vi "CH0_write_byte_data_into_mem.vi"(0 "MB data":u8, 1 "UB data":u8, 3 "USB Interface Name":refnum<visa-resource-name>="COM3", 4 "HB data":u8, 5 "LB data":u8, 6 "MB address":string, 7 "HB address":string, 9 "WRITE DATA":bool, 10 "Input buffer size":u32=16384, 11 "LB address":string, 12 "UB address":string, 13 "error in (no error)":errorcluster) -> (14 "MB data string":string, 15 "UB data string":string, 17 "error out":errorcluster, 18 "HB data string":string, 19 "LB data string":string)   [LabVIEW 2012]
panel:
  out "T command Bytes sent 4":dbl
  out "T command Bytes sent 3":dbl
  out "T command Bytes sent 2":dbl
  out "T command Bytes sent":dbl
  out "First 'T' Number of bytes written":dbl
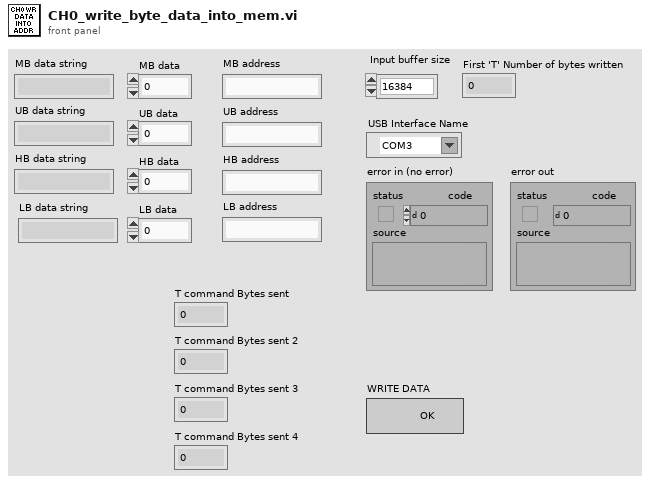
[diagram p1: front panel]
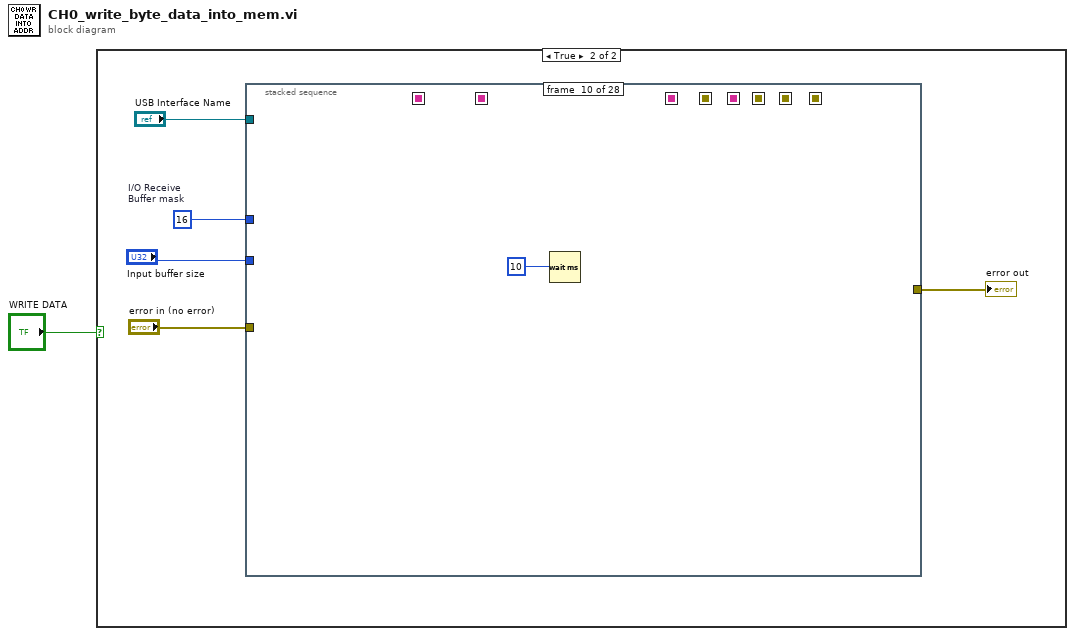
[diagram p0: block diagram]
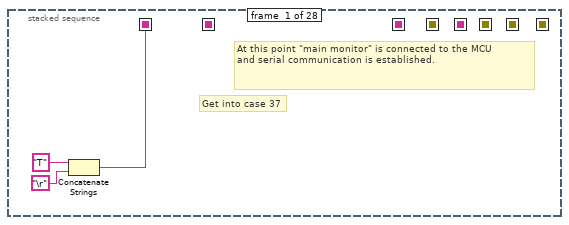
[diagram p3: hidden frame]
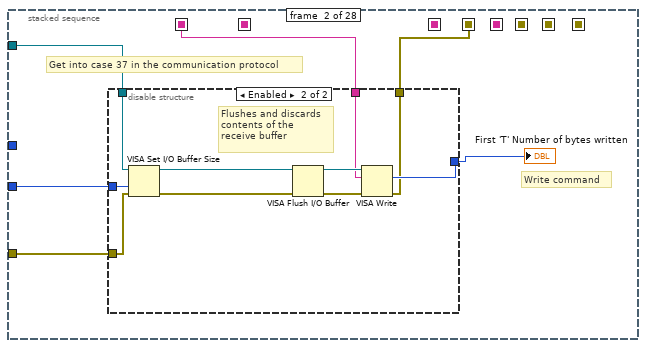
[diagram p4: hidden frame]
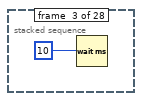
[diagram p6: hidden frame]
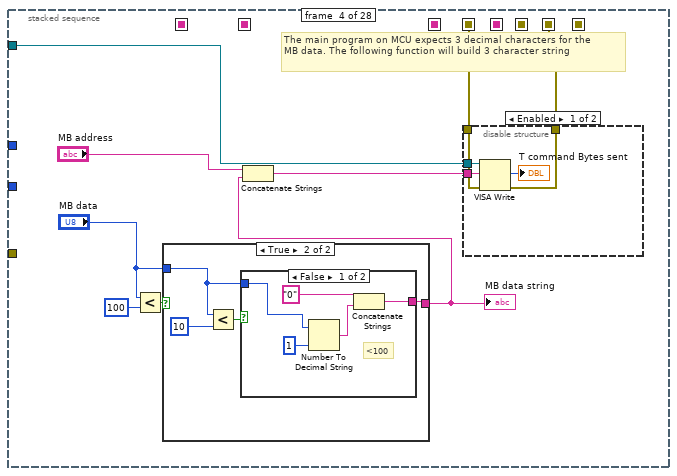
[diagram p7: hidden frame]
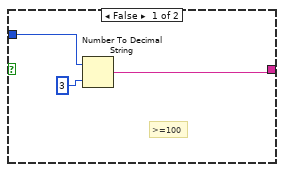
[diagram p8: hidden frame]
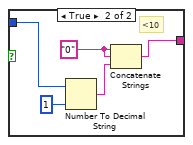
[diagram p9: hidden frame]
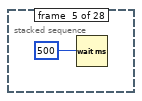
[diagram p11: hidden frame]
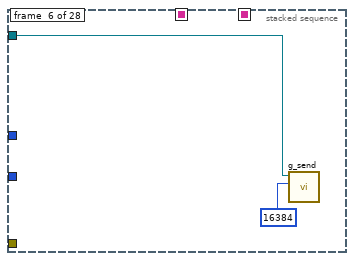
[diagram p12: hidden frame]
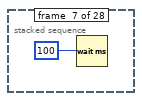
[diagram p13: hidden frame]
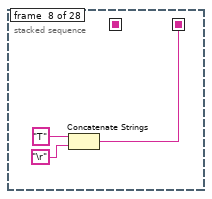
[diagram p14: hidden frame]
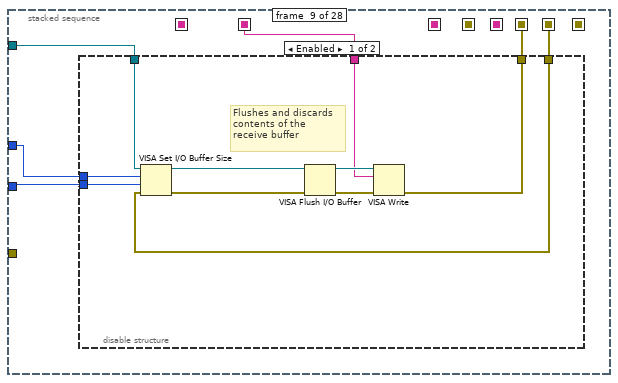
[diagram p15: hidden frame]
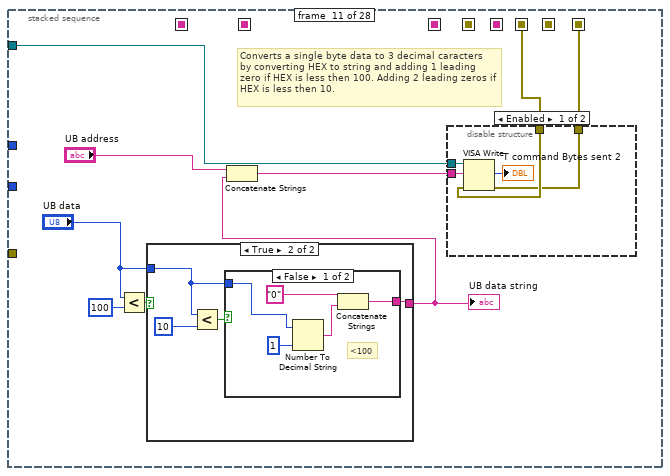
[diagram p17: hidden frame]
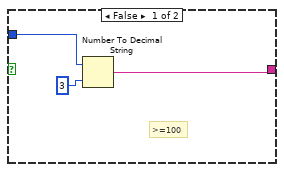
[diagram p18: hidden frame]
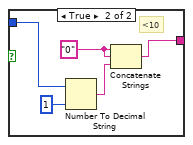
[diagram p19: hidden frame]
diagram:
  n1 = case shown="True" "WRITE DATA" {
    frame False {
    }
    frame True {
      w4 = u16 16  # I/O Receive Buffer mask
      n2 = stacked-sequence {
        seq-local: [w7 _ _ _ _ _ _ _ _ _ _ _ _ _ _ _ _ _ _ _ _ _ _ _ _ _ _ _] -> [_ w12 _ _ _ _ _ _ _ _ _ _ _ _ _ _ _ _ _ _ _ _ _ _ _ _ _ _]
        seq-local: [_ _ _ _ _ _ _ w62 _ _ _ _ _ _ _ _ _ _ _ _ _ _ _ _ _ _ _ _] -> [_ _ _ _ _ _ _ _ w67 _ _ _ _ _ _ _ _ _ _ _ _ _ _ _ _ _ _ _]
        seq-local: [_ _ _ _ _ _ _ _ _ _ _ _ _ _ w117 _ _ _ _ _ _ _ _ _ _ _ _ _] -> [_ _ _ _ _ _ _ _ _ _ _ _ _ _ _ w121 _ _ _ _ _ _ _ _ _ _ _ _]
        seq-local: [_ _ _ _ _ _ _ _ _ _ _ _ _ _ _ _ _ _ _ _ _ w166 _ _ _ _ _ _] -> [_ _ _ _ _ _ _ _ _ _ _ _ _ _ _ _ _ _ _ _ _ _ w169 _ _ _ _ _]
        seq-local: [_ w10 _ _ _ _ _ _ _ _ _ _ _ _ _ _ _ _ _ _ _ _ _ _ _ _ _ _] -> [_ _ _ w28 _ _ _ _ _ _ _ _ _ _ _ _ _ _ _ _ _ _ _ _ _ _ _ _]
        seq-local: [_ _ _ w27 _ _ _ _ _ _ _ _ _ _ _ _ _ _ _ _ _ _ _ _ _ _ _ _] -> [_ _ _ _ _ _ _ _ w66 _ _ _ _ _ _ _ _ _ _ _ _ _ _ _ _ _ _ _]
        seq-local: [_ _ _ _ _ _ _ _ w65 _ _ _ _ _ _ _ _ _ _ _ _ _ _ _ _ _ _ _] -> [_ _ _ _ _ _ _ _ _ _ w83 _ _ _ _ _ _ _ _ _ _ _ _ _ _ _ _ _]
        seq-local: [_ _ _ _ _ _ _ _ _ _ w82 _ _ _ _ _ _ _ _ _ _ _ _ _ _ _ _ _] -> [_ _ _ _ _ _ _ _ _ _ _ _ _ _ _ w120 _ _ _ _ _ _ _ _ _ _ _ _]
        tunnel: "USB Interface Name" -> [_ w15 _ w34 _ w59 _ _ w70 _ w85 _ w114 _ _ w124 _ w136 _ w163 _ _ w173 _ w187 _ w215 _]
        tunnel: "error in (no error)" -> [_ w14 _ _ _ _ _ _ _ _ _ _ _ _ _ _ _ _ _ _ _ _ w171 _ _ _ _ _]
        tunnel: "Input buffer size" -> [_ w13 _ _ _ _ _ _ w69 _ _ _ _ _ _ w122 _ _ _ _ _ _ w172 _ _ _ _ _]
        tunnel: w4 -> [_ _ _ _ _ _ _ _ w68 _ _ _ _ _ _ w123 _ _ _ _ _ _ w170 _ _ _ _ _]
        tunnel: [_ _ _ _ _ _ _ _ _ _ _ _ _ _ _ _ _ _ _ _ _ _ _ _ w185 _ _ _] -> w3
        frame #0 {
          # "At this point \"main monitor\" is connected to the MCU\nand serial communication is established."
          # "Get into case 37"
          n3 = Concatenate Strings("T", "\r") -> (w7:string)
        }
        frame #1 {
          # "Get into case 37 in the communication protocol"
          # "Write command"
          n4 = disable-structure shown="Enabled" {
            disable-tunnel: w13 -> [_ w21]
            disable-tunnel: w12 -> [_ w20]
            disable-tunnel: w15 -> [_ w19]
            disable-tunnel: w14 -> [_ w18]
            disable-tunnel: [_ w17] -> w11
            disable-tunnel: [_ w16] -> w10
            frame Disabled {
            }
            frame Enabled {
              # "Flushes and discards \ncontents of the \nreceive buffer"
              n5 = VISA Set I/O Buffer Size(VISA resource name=w19, size (4096)=w21, error in (no error)=w18) -> (VISA resource name out=w23:refnum<visa-resource-name>, error out=w22:errorcluster)  [unwired: 1 in]
              n6 = VISA Flush I/O Buffer(VISA resource name=w23, error in (no error)=w22) -> (VISA resource name out=w25:refnum<visa-resource-name>, error out=w24:errorcluster)  [unwired: 1 in]
              n7 = VISA Write(VISA resource name=w25, write buffer=w20, error in (no error)=w24) -> (return count=w17:u32, error out=w16:errorcluster)  [unwired: 1 out]
            }
          }
          "First 'T' Number of bytes written" <- w11
        }
        frame #2 {
          n8 = Wait (ms)(milliseconds to wait=10) -> ()  [unwired: 1 out]
        }
        frame #3 {
          # "The main program on MCU expects 3 decimal characters for the \nMB data. The following function will build 3 character string"
          n9 = Less?(x="MB data", y=100) -> (x < y?=w32:bool)
          n10 = case shown="True" w32 {
            tunnel: [w38 w39] -> w29
            tunnel: "MB data" -> [w36 w40]
            frame False {
              # ">=100"
              n11 = Number To Decimal String(number=w36, width (-)=3) -> (decimal integer string=w38:string)
            }
            frame True {
              n12 = Less?(x=w40, y=10) -> (x < y?=w42:bool)
              n13 = case shown="False" w42 {
                tunnel: w40 -> [w44 w48]
                tunnel: [w43 w49] -> w39
                frame False {
                  # "<100"
                  n14 = Number To Decimal String(number=w44, width (-)=1) -> (decimal integer string=w45:string)
                  n15 = Concatenate Strings("0", w45) -> (w43:string)
                }
                frame True {
                  w50 = "0"
                  # "<10"
                  n16 = Number To Decimal String(number=w48, width (-)=1) -> (decimal integer string=w51:string)
                  n17 = Concatenate Strings(w50, w50, w51) -> (w49:string)
                }
              }
            }
          }
          "MB data string" <- w29
          n18 = Concatenate Strings("MB address", w29) -> (w35:string)
          n19 = disable-structure shown="Enabled" {
            disable-tunnel: w35 -> [w56 _]
            disable-tunnel: w34 -> [w55 _]
            disable-tunnel: w28 -> [w54 _]
            disable-tunnel: [w53 _] -> w27
            frame Enabled {
              n20 = VISA Write(VISA resource name=w55, write buffer=w56, error in (no error)=w54) -> (return count=→"T command Bytes sent":u32, error out=w53:errorcluster)  [unwired: 1 out]
            }
            frame Disabled {
            }
          }
        }
        frame #4 {
          n21 = Wait (ms)(milliseconds to wait=500) -> ()  [unwired: 1 out]
        }
        frame #5 {
          n22 = call "g_send.vi"("Input buffer size"=16384, "USB Interface Name"=w59) -> ()  [unwired: 9 in, 1 out]
        }
        frame #6 {
          n23 = Wait (ms)(milliseconds to wait=100) -> ()  [unwired: 1 out]
        }
        frame #7 {
          n24 = Concatenate Strings("T", "\r") -> (w62:string)
        }
        frame #8 {
          n25 = disable-structure shown="Enabled" {
            disable-tunnel: w70 -> [w76 _]
            disable-tunnel: w69 -> [w75 _]
            disable-tunnel: w68 -> [w74 _]
            disable-tunnel: w67 -> [w73 _]
            disable-tunnel: w66 -> [w72 _]
            disable-tunnel: [w71 _] -> w65
            frame Enabled {
              # "Flushes and discards \ncontents of the \nreceive buffer"
              n26 = VISA Set I/O Buffer Size(VISA resource name=w76, mask (16)=w74, size (4096)=w75, error in (no error)=w72) -> (VISA resource name out=w78:refnum<visa-resource-name>, error out=w77:errorcluster)
              n27 = VISA Flush I/O Buffer(VISA resource name=w78, error in (no error)=w77) -> (VISA resource name out=w80:refnum<visa-resource-name>, error out=w79:errorcluster)  [unwired: 1 in]
              n28 = VISA Write(VISA resource name=w80, write buffer=w73, error in (no error)=w79) -> (error out=w71:errorcluster)  [unwired: 2 out]
            }
            frame Disabled {
            }
          }
        }
        frame #9 {
          n29 = Wait (ms)(milliseconds to wait=10) -> ()  [unwired: 1 out]
        }
        frame #10 {
          # "Converts a single byte data to 3 decimal caracters\nby converting HEX to string and adding 1 leading zero if HEX is less then 100. Adding 2 leading zeros if HEX is less then 10."
          n30 = Less?(x="UB data", y=100) -> (x < y?=w89:bool)
          n31 = case shown="True" w89 {
            tunnel: [w93 w94] -> w86
            tunnel: "UB data" -> [w91 w95]
            frame False {
              # ">=100"
              n32 = Number To Decimal String(number=w91, width (-)=3) -> (decimal integer string=w93:string)
            }
            frame True {
              n33 = Less?(x=w95, y=10) -> (x < y?=w97:bool)
              n34 = case shown="False" w97 {
                tunnel: w95 -> [w99 w103]
                tunnel: [w98 w104] -> w94
                frame False {
                  # "<100"
                  n35 = Number To Decimal String(number=w99, width (-)=1) -> (decimal integer string=w100:string)
                  n36 = Concatenate Strings("0", w100) -> (w98:string)
                }
                frame True {
                  w105 = "0"
                  # "<10"
                  n37 = Number To Decimal String(number=w103, width (-)=1) -> (decimal integer string=w106:string)
                  n38 = Concatenate Strings(w105, w105, w106) -> (w104:string)
                }
              }
            }
          }
          "UB data string" <- w86
          n39 = Concatenate Strings("UB address", w86) -> (w90:string)
          n40 = disable-structure shown="Enabled" {
            disable-tunnel: w90 -> [w111 _]
            disable-tunnel: w85 -> [w110 _]
            disable-tunnel: w83 -> [w109 _]
            disable-tunnel: [w108 _] -> w82
            frame Enabled {
              n41 = VISA Write(VISA resource name=w110, write buffer=w111, error in (no error)=w109) -> (return count=→"T command Bytes sent 2":u32, error out=w108:errorcluster)  [unwired: 1 out]
            }
            frame Disabled {
            }
          }
        }
        frame #11 {
          n42 = Wait (ms)(milliseconds to wait=500) -> ()  [unwired: 1 out]
        }
        frame #12 {
          n43 = call "g_send.vi"("Input buffer size"=16384, "USB Interface Name"=w114) -> ()  [unwired: 9 in, 1 out]
        }
        frame #13 {
          n44 = Wait (ms)(milliseconds to wait=100) -> ()  [unwired: 1 out]
        }
        frame #14 {
          n45 = Concatenate Strings("T", "\r") -> (w117:string)
        }
        frame #15 {
          n46 = disable-structure shown="Enabled" {
            disable-tunnel: w124 -> [w129 _]
            disable-tunnel: w123 -> [w128 _]
            disable-tunnel: w122 -> [w127 _]
            disable-tunnel: w121 -> [w126 _]
            disable-tunnel: w120 -> [w125 _]
            frame Enabled {
              # "Flushes and discards \ncontents of the \nreceive buffer"
              n47 = VISA Set I/O Buffer Size(VISA resource name=w129, mask (16)=w128, size (4096)=w127, error in (no error)=w125) -> (VISA resource name out=w131:refnum<visa-resource-name>, error out=w130:errorcluster)
              n48 = VISA Flush I/O Buffer(VISA resource name=w131, error in (no error)=w130) -> (VISA resource name out=w133:refnum<visa-resource-name>, error out=w132:errorcluster)  [unwired: 1 in]
              n49 = VISA Write(VISA resource name=w133, write buffer=w126, error in (no error)=w132) -> ()  [unwired: 3 out]
            }
            frame Disabled {
            }
          }
        }
        frame #16 {
          n50 = Wait (ms)(milliseconds to wait=10) -> ()  [unwired: 1 out]
        }
        frame #17 {
          # "Converts a single byte data to 3 decimal caracters\nby converting HEX to string and adding 1 leading zero if HEX is less then 100. Adding 2 leading zeros if HEX is less then 10."
          n51 = Less?(x="HB data", y=100) -> (x < y?=w140:bool)
          n52 = case shown="True" w140 {
            tunnel: [w144 w145] -> w137
            tunnel: "HB data" -> [w142 w146]
            frame False {
              # ">=100"
              n53 = Number To Decimal String(number=w142, width (-)=3) -> (decimal integer string=w144:string)
            }
            frame True {
              n54 = Less?(x=w146, y=10) -> (x < y?=w148:bool)
              n55 = case shown="False" w148 {
                tunnel: w146 -> [w150 w154]
                tunnel: [w149 w155] -> w145
                frame False {
                  # "<100"
                  n56 = Number To Decimal String(number=w150, width (-)=1) -> (decimal integer string=w151:string)
                  n57 = Concatenate Strings("0", w151) -> (w149:string)
                }
                frame True {
                  w156 = "0"
                  # "<10"
                  n58 = Number To Decimal String(number=w154, width (-)=1) -> (decimal integer string=w157:string)
                  n59 = Concatenate Strings(w156, w156, w157) -> (w155:string)
                }
              }
            }
          }
          "HB data string" <- w137
          n60 = Concatenate Strings("HB address", w137) -> (w141:string)
          n61 = disable-structure shown="Enabled" {
            disable-tunnel: w141 -> [w160 _]
            disable-tunnel: w136 -> [w159 _]
            frame Enabled {
              n62 = VISA Write(VISA resource name=w159, write buffer=w160) -> (return count=→"T command Bytes sent 3":u32)  [unwired: 1 in, 2 out]
            }
            frame Disabled {
            }
          }
        }
        frame #18 {
          n63 = Wait (ms)(milliseconds to wait=500) -> ()  [unwired: 1 out]
        }
        frame #19 {
          n64 = call "g_send.vi"("Input buffer size"=16384, "USB Interface Name"=w163) -> ()  [unwired: 9 in, 1 out]
        }
        frame #20 {
          n65 = Wait (ms)(milliseconds to wait=100) -> ()  [unwired: 1 out]
        }
        frame #21 {
          # "Get into case 37"
          n66 = Concatenate Strings("T", "\r") -> (w166:string)
        }
        frame #22 {
          # "Get into case 37 in the communication protocol"
          # "Write command"
          n67 = disable-structure shown="Enabled" {
            disable-tunnel: w172 -> [w179 _]
            disable-tunnel: w169 -> [w178 _]
            disable-tunnel: w173 -> [w177 _]
            disable-tunnel: w171 -> [w176 _]
            disable-tunnel: [w175 _] -> _
            disable-tunnel: w170 -> [w174 _]
            frame Enabled {
              # "Flushes and discards \ncontents of the \nreceive buffer"
              n68 = VISA Set I/O Buffer Size(VISA resource name=w177, mask (16)=w174, size (4096)=w179, error in (no error)=w176) -> (VISA resource name out=w181:refnum<visa-resource-name>, error out=w180:errorcluster)
              n69 = VISA Flush I/O Buffer(VISA resource name=w181, error in (no error)=w180) -> (VISA resource name out=w183:refnum<visa-resource-name>, error out=w182:errorcluster)  [unwired: 1 in]
              n70 = VISA Write(VISA resource name=w183, write buffer=w178, error in (no error)=w182) -> (return count=w175:u32)  [unwired: 2 out]
            }
            frame Disabled {
            }
          }
        }
        frame #23 {
          n71 = Wait (ms)(milliseconds to wait=10) -> ()  [unwired: 1 out]
        }
        frame #24 {
          # "The main program on MCU expects 3 decimal characters for the \nMB data. The following function will build 3 character string"
          n72 = Less?(x="LB data", y=100) -> (x < y?=w191:bool)
          n73 = case shown="True" w191 {
            tunnel: [w195 w196] -> w188
            tunnel: "LB data" -> [w193 w197]
            frame False {
              # ">=100"
              n74 = Number To Decimal String(number=w193, width (-)=3) -> (decimal integer string=w195:string)
            }
            frame True {
              n75 = Less?(x=w197, y=10) -> (x < y?=w199:bool)
              n76 = case shown="False" w199 {
                tunnel: w197 -> [w201 w205]
                tunnel: [w200 w206] -> w196
                frame False {
                  # "<100"
                  n77 = Number To Decimal String(number=w201, width (-)=1) -> (decimal integer string=w202:string)
                  n78 = Concatenate Strings("0", w202) -> (w200:string)
                }
                frame True {
                  w207 = "0"
                  # "<10"
                  n79 = Number To Decimal String(number=w205, width (-)=1) -> (decimal integer string=w208:string)
                  n80 = Concatenate Strings(w207, w207, w208) -> (w206:string)
                }
              }
            }
          }
          "LB data string" <- w188
          n81 = Concatenate Strings("LB address", w188) -> (w192:string)
          n82 = disable-structure shown="Enabled" {
            disable-tunnel: w192 -> [w212 _]
            disable-tunnel: w187 -> [w211 _]
            disable-tunnel: [w210 _] -> w185
            frame Enabled {
              n83 = VISA Write(VISA resource name=w211, write buffer=w212) -> (return count=→"T command Bytes sent 4":u32, error out=w210:errorcluster)  [unwired: 1 in, 1 out]
            }
            frame Disabled {
            }
          }
        }
        frame #25 {
          n84 = Wait (ms)(milliseconds to wait=500) -> ()  [unwired: 1 out]
        }
        frame #26 {
          n85 = call "g_send.vi"("Input buffer size"=16384, "USB Interface Name"=w215) -> ()  [unwired: 9 in, 1 out]
        }
        frame #27 {
          n86 = Wait (ms)(milliseconds to wait=100) -> ()  [unwired: 1 out]
        }
      }
      "error out" <- w3
    }
  }
